vi "Read Driver Status.vi"(8 "error in (no error)":errorcluster, 11 "Driver in":refnum<class "Driver.lvclass">) -> (0 "error out":errorcluster, 2 "Driver Status":T1 {"Current Xbox Controller"."Right Joystick"."Right" min=-1.0 max=1.0 step=0.1 scale=-1.0..1.0; "Current Xbox Controller"."Right Joystick"."Forward" min=-1.0 max=1.0 step=0.1 scale=-1.0..1.0; "Current Xbox Controller"."Left Joystick"."Right" min=-1.0 max=1.0 step=0.1 scale=-1.0..1.0; "Current Xbox Controller"."Left Joystick"."Forward" min=-1.0 max=1.0 step=0.1 scale=-1.0..1.0}, 3 "Driver out":refnum<class "Driver.lvclass">)   [LabVIEW 2013, in "Logical Systems.lvlib" / "Driver.lvlib" / "Driver.lvclass"]
uses:
  Driver.lvclass
  Driver Status.ctl
  XBox Controller/Xbox Controller.ctl
  Virtual Systems/XBox Controller/XBox Controller Class/Joystick.ctl
  Driver.lvclass/Driver.ctl
  XBox Controller/XBox Controller Class/Xbox Controller.lvlib
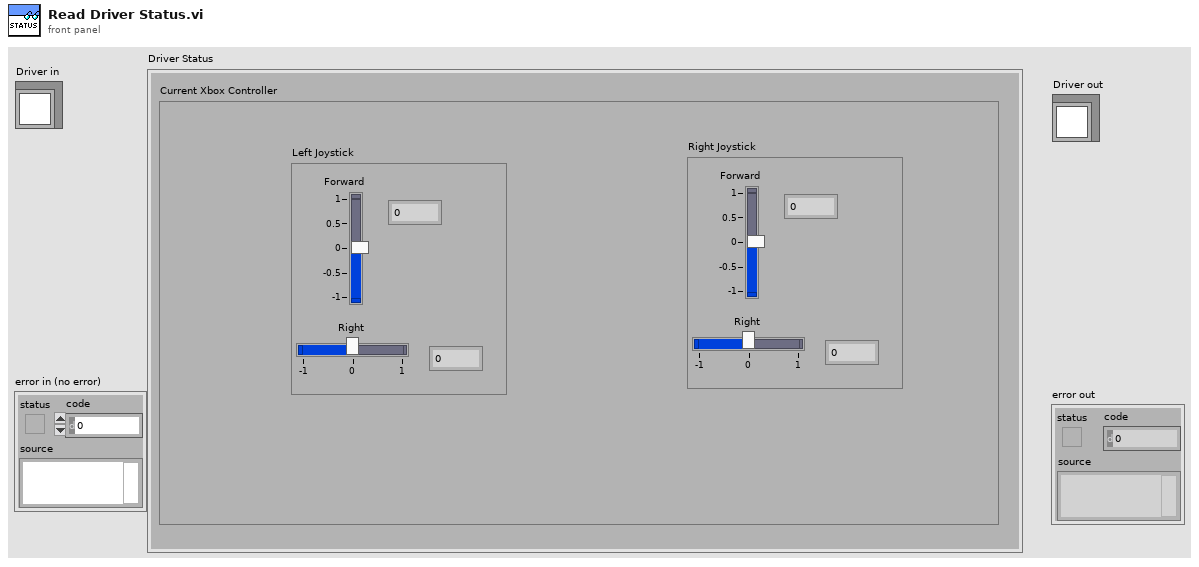
[diagram p1: front panel]
types:
  T1 = typedef "Logical Systems.lvlib/Driver.lvlib/Driver.lvclass/Driver Status.ctl" = cluster{"Current Xbox Controller":T2}
  T2 = typedef "Logical Systems.lvlib/Xbox Controller.lvlib/Xbox Controller.ctl" = cluster{"Left Joystick":T3, "Right Joystick":T3}
  T3 = typedef "Logical Systems.lvlib/Xbox Controller.lvlib/Joystick.ctl" = cluster{"Forward":dbl, "Right":dbl}
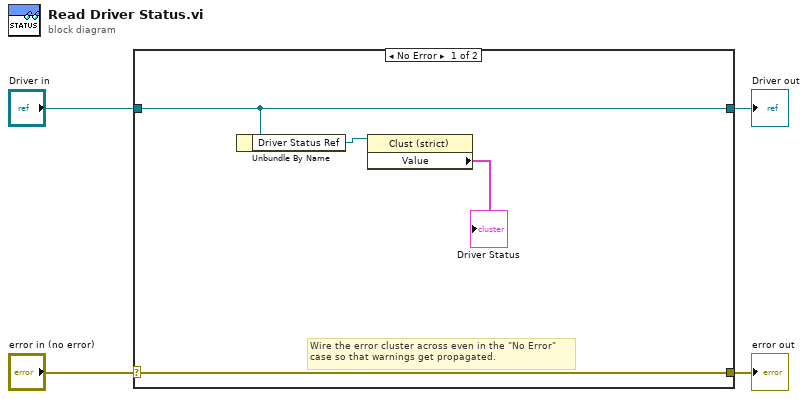
[diagram p0: block diagram]
diagram:
  n1 = case shown="No Error" "error in (no error)" {
    selector: "error in (no error)" -> [w8 w10]
    tunnel: [w8 w10] -> w3
    tunnel: [w7 w9] -> w1
    tunnel: "Driver in" -> [w7 w9]
    frame No Error {
      # "Wire the error cluster across even in the \"No Error\"\ncase so that warnings get propagated."
      n2 = Unbundle By Name(w7) -> ("Driver Status Ref"=w6:refnum<vi>)
      n3 = property class="Clust (strict)"(reference=w6) -> ("Value"=→"Driver Status":cluster{"Current Xbox Controller":T2})  [unwired: 1 in, 2 out]
    }
    frame Error {
    }
  }
  "error out" <- w3
  "Driver out" <- w1
